vi "Set primaryFixedDim.vi"(8 "error in":errorcluster, 10 "primaryFixedDim":u32(colorbox), 11 "Material-Scheme in":refnum<class "Material-Scheme.lvclass">) -> (0 "error out":errorcluster, 3 "Material-Scheme out":refnum<class "Material-Scheme.lvclass">)   [LabVIEW 2026, in "TSC Material Theme.lvlib" / "Material-Scheme.lvclass"]
doc: "set the color for: primaryFixedDim\n\n<b>Code Developed By:</b> +\nDaniel Coons +\nTechnology Service Corporation +\nwww.tsc.com/atcs"
uses:
  Material-Scheme.lvclass
  Material-Scheme.lvclass/Material-Scheme.ctl
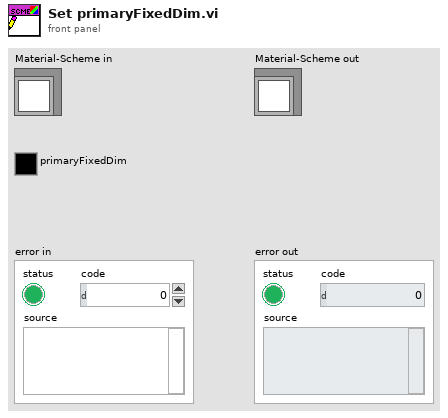
[diagram p1: front panel]
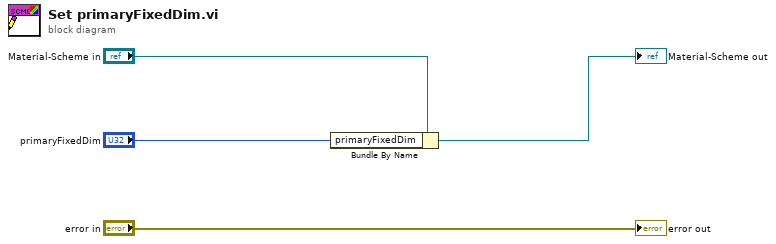
[diagram p0: block diagram]
diagram:
  n1 = Bundle By Name(cluster="Material-Scheme in", "primaryFixedDim"="primaryFixedDim") -> (→"Material-Scheme out":refnum<class "Material-Scheme.lvclass">)
  "error out" <- "error in"
